vi "Logging Build Tree.vi"(5 "Entries":T1, 7 "TreeRef":refnum<vi>) -> (3 "TreeRef":refnum<vi>)   [LabVIEW 2012, in "femtoRoboLib.lvlib"]
uses:
  femtoRoboLib.lvlib
  Log Entry Block.ctl
  Log Entry.ctl
  Log Value Type.ctl
  Log Value Cluster.ctl
panel:
  out "All Tags":string[](array[string])
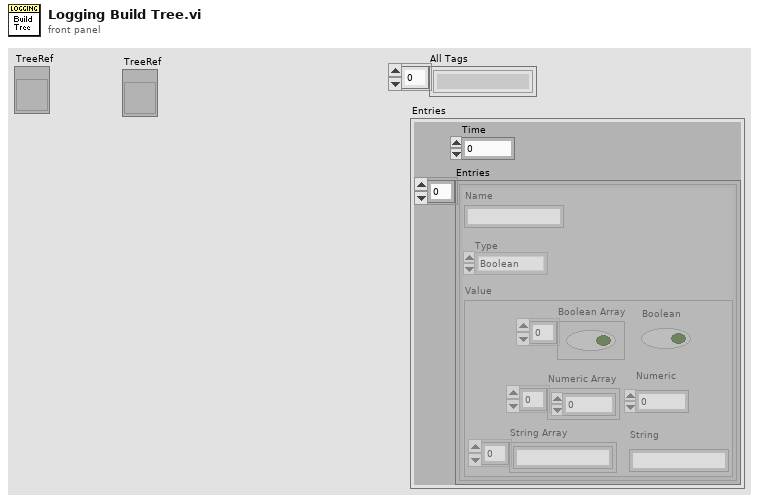
[diagram p1: front panel]
types:
  T1 = typedef "femtoRoboLib.lvlib/Log Entry Block.ctl" = cluster{"Entries":T2[], "Time":u32}
  T2 = typedef "femtoRoboLib.lvlib/Log Entry.ctl" = cluster{"Name":string, "Type":T3, "Value":T4}
  T3 = typedef "femtoRoboLib.lvlib/Log Value Type.ctl" = enum16{"Boolean", "Numeric", "String", "Boolean Array", "Numeric Array", "String Array"}
  T4 = typedef "femtoRoboLib.lvlib/Log Value Cluster.ctl" = cluster{"Boolean Array":bool[], "Boolean":bool, "Numeric Array":dbl[], "Numeric":dbl, "String Array":string[], "String":string}
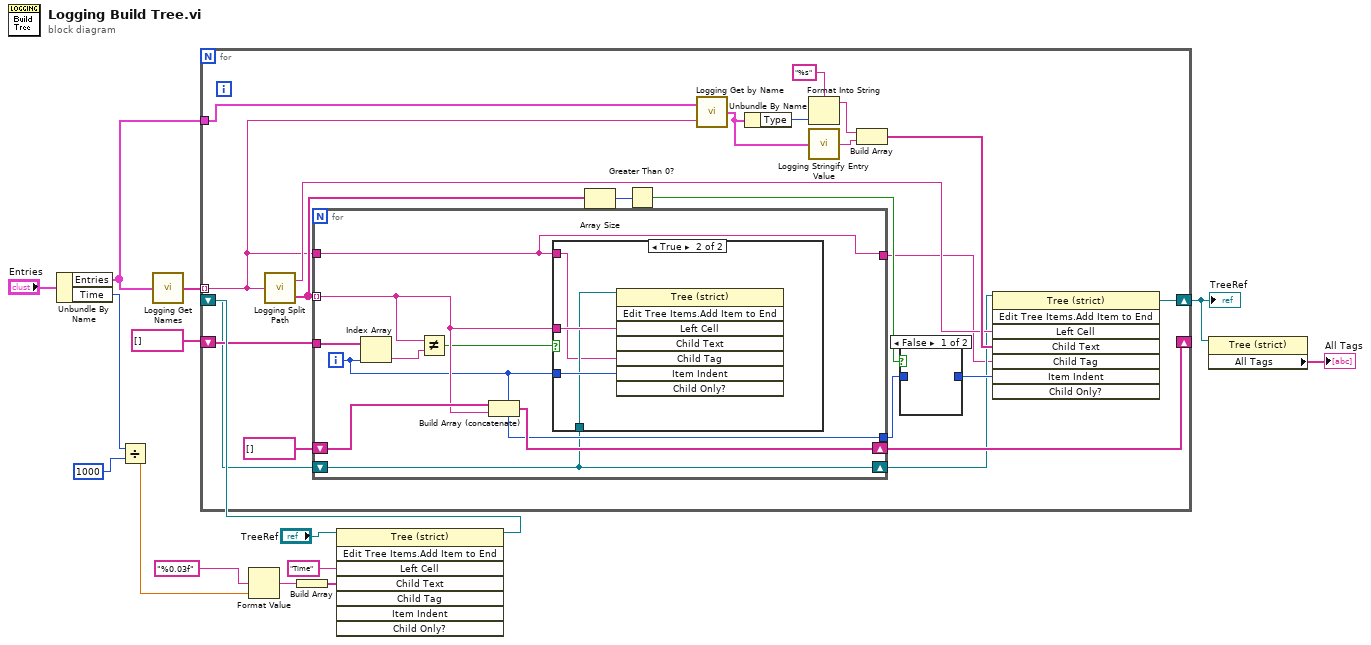
[diagram p0: block diagram]
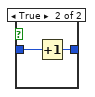
[diagram p2: hidden frame]
diagram:
  n1 = Unbundle By Name("Entries") -> ("Entries"=w12:T2[], "Time"=w6:u32)
  n2 = Divide(x=w6, y=u32 1000) -> (x/y=w5:dbl)
  n3 = call "Logging Get Names.vi"("Entries"=w12) -> ("Names"=w15:string[])
  n4 = Format Value(format string="%0.03f", value (0)=w5) -> (output string=w9:string)  [unwired: 1 in]
  n5 = Build Array(w9) -> (w8:string[])
  n6 = invoke class="Tree (strict)" method="Edit Tree Items.Add Item to End"(reference="TreeRef", "Left Cell"="Time" ("Left Cell String"), "Child Text"=w8) -> (reference out=w2:refnum<vi>)  [unwired: 5 in, 7 out]
  n7 = for {
    tunnel: w15 -> [w19] mode=indexing
    shift-right: [w34] -> _
    shift-left: string[] [] ("Split Path") -> [w36]
    tunnel: w12 -> [w33]
    shift-right: [w17] -> w1
    shift-left: w2 -> [w16]
    n8 = call "Logging Split Path.vi"("Path In"=w19) -> ("Name"=w24:string, "Split Path"=w21:string[])
    n9 = for {
      tunnel: w21 -> [w43] mode=indexing
      tunnel: w36 -> [w47]
      shift-right: [w45] -> w34
      shift-left: string[] [] -> [w44]
      tunnel: [w41] -> w25
      shift-right: [w40] -> w23
      shift-left: w16 -> [w40]
      tunnel: w19 -> [w39]
      tunnel: [w39] -> w18
      i -> [w41]
      n10 = Index Array(array=w47, index=w41) -> (element=w46:string)
      n11 = Not Equal?(x=w43, y=w46) -> (x != y?=w42:bool)
      n12 = Build Array (concatenate)(w44, w43) -> (w45:string[])
      n13 = case shown="True" w42 {
        tunnel: w43 -> [_ w51]
        tunnel: w41 -> [_ w50]
        tunnel: w40 -> [_ w49]
        tunnel: w39 -> [_ w48]
        frame False {
        }
        frame True {
          n14 = invoke class="Tree (strict)" method="Edit Tree Items.Add Item to End"(reference=w49, "Left Cell"=w51, "Child Tag"=w48, "Item Indent"=w50) -> ()  [unwired: 4 in, 8 out]
        }
      }
    }
    n15 = Array Size(array=w21) -> (size(s)=w22:i32)
    n16 = Greater Than 0?(x=w22) -> (x > 0?=w20:bool)
    n17 = call "Logging Get by Name.vi"("Name"=w19, "Entries"=w33) -> ("Entry"=w29:T2)
    n18 = Unbundle By Name(w29) -> ("Type"=w31:T3)
    n19 = Format Into String(format string="%s", w31) -> (resulting string=w30:string)  [unwired: 2 in, 1 out]
    n20 = call "Logging Stringify Entry Value.vi"("Entry"=w29) -> ("String"=w28:string)
    n21 = Build Array(w30, w28) -> (w27:string[])
    n22 = case shown="False" w20 {
      tunnel: [_ w38] -> w26
      tunnel: w25 -> [_ w37]
      frame False {
      }
      frame True {
        n23 = Increment(x=w37) -> (x+1=w38:i32)
      }
    }
    n24 = invoke class="Tree (strict)" method="Edit Tree Items.Add Item to End"(reference=w23, "Left Cell"=w24, "Child Text"=w27, "Child Tag"=w18, "Item Indent"=w26) -> (reference out=w17:refnum<vi>)  [unwired: 3 in, 7 out]
  }
  "TreeRef" <- w1
  n25 = property class="Tree (strict)"(reference=w1) -> ("All Tags"=→"All Tags":string[])  [unwired: 1 in, 2 out]
